vi "Levelmeter_Queue_Commands.vi"(1 "Mischer Levelmeter  Control":T1={"N-Shield Refill"=FALSE, "Automatic Refill Shield"=TRUE, "Trap Refill"=FALSE, "Automatic Refill Trap"=TRUE}, 3 "Mischer Levelmeter N":refnum<queue>) -> (0 "New Status":T1={"N-Shield Refill"=FALSE, "Automatic Refill Shield"=TRUE, "Trap Refill"=FALSE, "Automatic Refill Trap"=TRUE})   [LabVIEW 2019]
uses:
  Mischer/Mischer_Levelmeter_Control.ctl
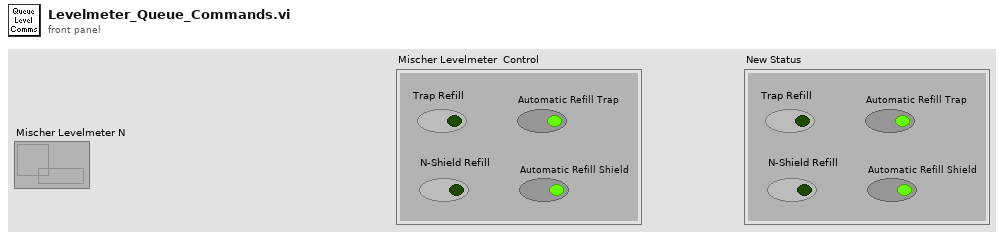
[diagram p1: front panel]
types:
  T1 = typedef "Mischer_Levelmeter_Control.ctl" = cluster{"N-Shield Refill":bool, "Automatic Refill Shield":bool, "Trap Refill":bool, "Automatic Refill Trap":bool}
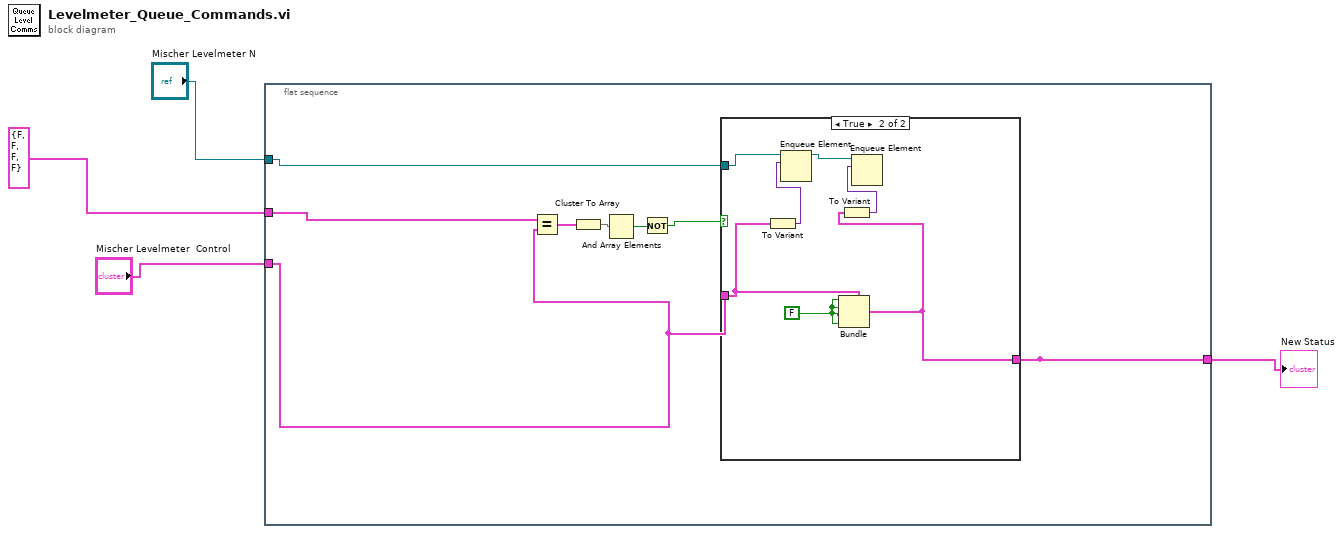
[diagram p0: block diagram]
diagram:
  n1 = flat-sequence {
    tunnel: "Mischer Levelmeter N" -> [w8]
    tunnel: T1 {"N-Shield Refill"=FALSE, "Automatic Refill Shield"=FALSE, "Trap Refill"=FALSE, "Automatic Refill Trap"=FALSE} ("Old Status") -> [w7]
    tunnel: "Mischer Levelmeter  Control" -> [w5]
    tunnel: [w6] -> _
    tunnel: [w6] -> w2
    frame #0 {
      n2 = Equal?(x=w7, y=w5) -> (x = y?=w12:T1)
      n3 = Cluster To Array(cluster=w12) -> (array=w11:bool[])
      n4 = And Array Elements(Boolean array=w11) -> (logical AND=w10:bool)
      n5 = Not(x=w10) -> (.not. x?=w9:bool)
      n6 = case shown="True" w9 {
        tunnel: w8 -> [_ w20]
        tunnel: w5 -> [w13 w17]
        tunnel: [w13 w15] -> w6
        frame False {
        }
        frame True {
          w14 = FALSE
          n7 = To Variant(anything=w17) -> (Variant=w19:variant)
          n8 = Enqueue Element(queue=w20, element=w19) -> (queue out=w18:refnum<queue>)  [unwired: 2 in, 2 out]
          n9 = Bundle(cluster=w17, "N-Shield Refill"=w14, "Automatic Refill Shield"=w14, "Trap Refill"=w14, "Automatic Refill Trap"=w14) -> (w15:T1)
          n10 = To Variant(anything=w15) -> (Variant=w16:variant)
          n11 = Enqueue Element(queue=w18, element=w16) -> ()  [unwired: 2 in, 3 out]
        }
      }
    }
  }
  "New Status" <- w2
